vi "Bottom_left_scanframe_coords.vi"(4 "error in":errorcluster, 7 "Application ref in":refnum<vi>) -> (0 "error out":errorcluster, 1 "Y_bl":sgl, 2 "X_bl":sgl, 3 "Application ref out":refnum<vi>)   [LabVIEW 2025]
uses:
  <userlib>/Nanonis Prog Interface V5/Nanonis Prog Interface.lvlib
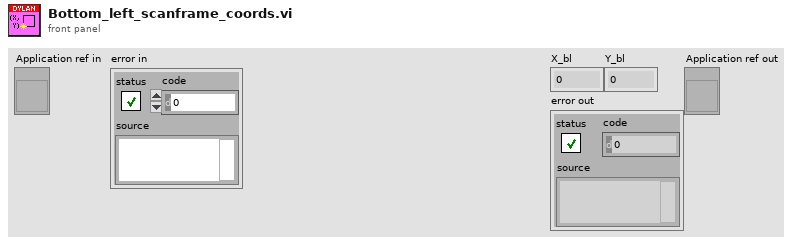
[diagram p1: front panel]
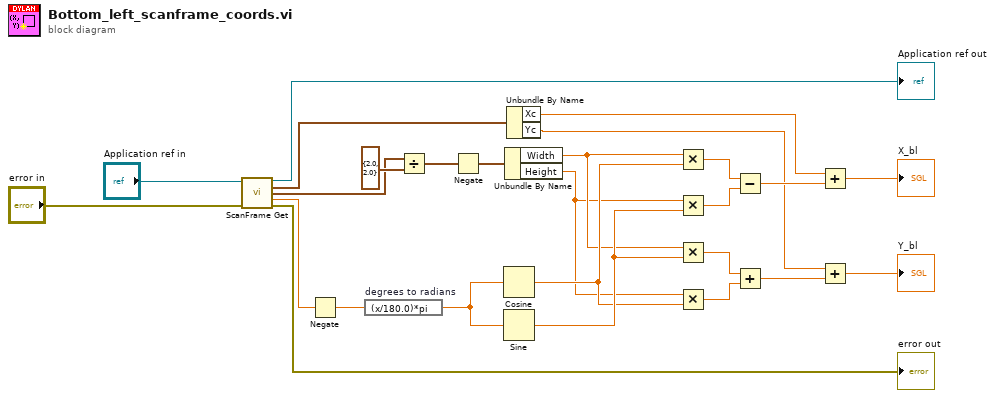
[diagram p0: block diagram]
diagram:
  n1 = call <userlib>:"ScanFrame Get.vi"("Application ref in"="Application ref in", "error in (no error)"="error in") -> ("Application ref out"=→"Application ref out":refnum<vi>, "Center coordinates (m)"=w25:cluster{"Xc":sgl, "Yc":sgl}, "Size (m)"=w24:cluster{"Width":sgl, "Height":sgl}, "Angle (deg)"=w20:sgl, "error out"=→"error out":errorcluster)  [unwired: 9 in]
  n2 = Negate(x=w20) -> (-x=w19:sgl)
  n3 = expression code="(x/180.0)*pi" "degrees to radians"(w19) -> (w21:sgl)
  n4 = Divide(x=w24, y=cluster{"Width":sgl, "Height":sgl} {"Width"=2.0, "Height"=2.0}) -> (x/y=w4:cluster{"Width":sgl, "Height":sgl})
  n5 = Negate(x=w4) -> (-x=w3:cluster{"Width":sgl, "Height":sgl})
  n6 = Cosine(x=w21) -> (cos(x)=w15:sgl)
  n7 = Sine(x=w21) -> (sin(x)=w16:sgl)
  n8 = Unbundle By Name(w3) -> ("Width"=w2:sgl, "Height"=w1:sgl)
  n9 = Unbundle By Name(w25) -> ("Xc"=w10:sgl, "Yc"=w7:sgl)
  n10 = Multiply(x=w2, y=w15) -> (x*y=w14:sgl)
  n11 = Multiply(x=w1, y=w16) -> (x*y=w13:sgl)
  n12 = Multiply(x=w2, y=w16) -> (x*y=w12:sgl)
  n13 = Multiply(x=w1, y=w15) -> (x*y=w11:sgl)
  n14 = Subtract(x=w14, y=w13) -> (x-y=w9:sgl)
  n15 = Add(x=w12, y=w11) -> (x+y=w8:sgl)
  n16 = Add(x=w10, y=w9) -> (x+y=→"X_bl":sgl)
  n17 = Add(x=w7, y=w8) -> (x+y=→"Y_bl":sgl)
